vi "Calc Increment_modded.vi"(1 "desired font(Application)":T5(ring)=enum."Application Font", 2 "scale definition":T2={"coordinate 1"=5, "value 1"=5.0, "coordinate 2"=5, "value 2"=5.0, "log"=FALSE, "fmt and prec"={"format"=enum."Hex", "precision"=0}} {"value 2" format="%0.2f"; "value 1" format="%0.2f"}, 3 "scale attributes":T3={"horizontal"=TRUE, "left/top"=FALSE, "draw bar"=FALSE, "line color"=0, "text color"=0}, 5 "[user-specified font]":T4) -> (6 "start":dbl format="%0.2f", 7 "increment":dbl format="%0.2f", 9 "text size":i16)   [LabVIEW 2018]
uses:
  fmt_prec_modded.ctl
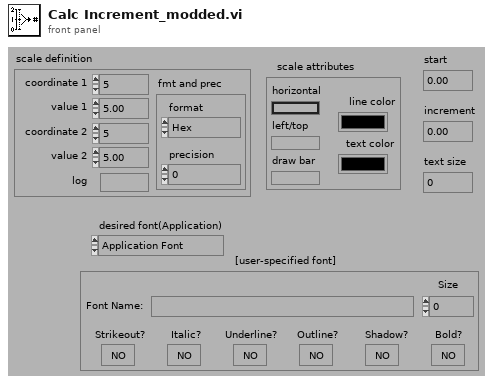
[diagram p1: front panel]
types:
  T1 = typedef "fmt_prec_modded.ctl" = cluster{"format":enum8{"Decimal", "Scientific", "Engineering", "Binary", "Octal", "Hex", "Timestamp"}, "precision":u8}
  T2 = cluster{"coordinate 1":i16, "value 1":dbl, "coordinate 2":i16, "value 2":dbl, "log":bool, "fmt and prec":T1}
  T3 = cluster{"horizontal":bool, "left/top":bool, "draw bar":bool, "line color":u32, "text color":u32}
  T4 = cluster{"Font Name:":string, "Size":i16, "Strikeout?":bool, "Italic?":bool, "Underline?":bool, "Outline?":bool, "Shadow?":bool, "Bold?":bool}
  T5 = enum16{"User-specified Font", "Application Font", "System Font", "Dialog Font"}
  T6 = cluster{"left":i16, "top":i16, "right":i16, "bottom":i16}
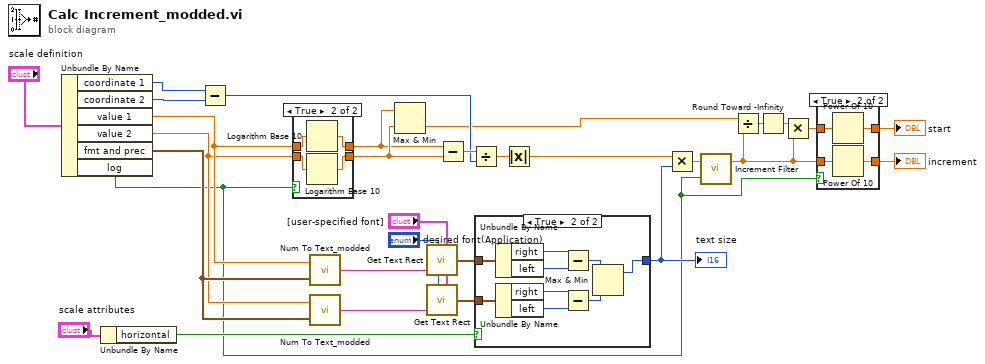
[diagram p0: block diagram]
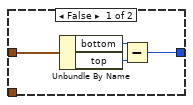
[diagram p4: hidden frame]
diagram:
  n1 = Unbundle By Name("scale definition") -> ("coordinate 1"=w14:i16, "coordinate 2"=w15:i16, "value 1"=w8:dbl, "value 2"=w7:dbl, "fmt and prec"=w28:T1, "log"=w1:bool)
  n2 = Unbundle By Name("scale attributes") -> ("horizontal"=w23:bool)
  n3 = Subtract(x=w14, y=w15) -> (x-y=w16:i16)
  n4 = case shown="True" w1 {
    tunnel: w8 -> [w32 w35]
    tunnel: [w32 w34] -> w10
    tunnel: w7 -> [w31 w36]
    tunnel: [w31 w33] -> w11
    frame False {
    }
    frame True {
      n5 = Logarithm Base 10(1:w35) -> (0:w34:dbl)
      n6 = Logarithm Base 10(1:w36) -> (0:w33:dbl)
    }
  }
  n7 = call "Num To Text_modded.vi"("fmt and prec"=w28, "number"=w8) -> ("numeric string"=w30:string)
  n8 = call "Num To Text_modded.vi"("fmt and prec"=w28, "number"=w7) -> ("numeric string"=w27:string)
  n9 = Max & Min(x=w10, y=w11) -> (min(x,y)=w9:dbl)  [unwired: 1 out]
  n10 = call <vilib>:"Get Text Rect.vi"("desired font(Application)"="desired font(Application)", "text"=w30, "[user-specified font]"="[user-specified font]") -> ("rect"=w21:T6)  [unwired: 6 in]
  n11 = call <vilib>:"Get Text Rect.vi"("desired font(Application)"="desired font(Application)", "text"=w27, "[user-specified font]"="[user-specified font]") -> ("rect"=w22:T6)  [unwired: 6 in]
  n12 = Subtract(x=w10, y=w11) -> (x-y=w18:dbl)
  n13 = Divide(x=w18, y=w16) -> (x/y=w20:dbl)
  n14 = case shown="True" w23 {
    tunnel: w22 -> [_ w48]
    tunnel: w21 -> [w38 w49]
    tunnel: [w37 w41] -> w17
    frame False {
      n15 = Unbundle By Name(w38) -> ("bottom"=w39:i16, "top"=w40:i16)
      n16 = Subtract(x=w39, y=w40) -> (x-y=w37:i16)
    }
    frame True {
      n17 = Unbundle By Name(w49) -> ("right"=w44:i16, "left"=w45:i16)
      n18 = Unbundle By Name(w48) -> ("right"=w47:i16, "left"=w46:i16)
      n19 = Subtract(x=w44, y=w45) -> (x-y=w42:i16)
      n20 = Subtract(x=w47, y=w46) -> (x-y=w43:i16)
      n21 = Max & Min(x=w42, y=w43) -> (max(x,y)=w41:i16)  [unwired: 1 out]
    }
  }
  "text size" <- w17
  n22 = Absolute Value(x=w20) -> (abs(x)=w19:dbl)
  n23 = Multiply(x=w19, y=w17) -> (x*y=w2:dbl)
  n24 = call <vilib>:"Increment Filter.vi"("log?(F)"=w1, "initial increment"=w2) -> ("nice increment"=w5:dbl)  [unwired: 1 in]
  n25 = Divide(x=w9, y=w5) -> (x/y=w13:dbl)
  n26 = Round Toward -Infinity(1:w13) -> (0:w12:dbl)
  n27 = Multiply(x=w12, y=w5) -> (x*y=w4:dbl)
  n28 = case shown="True" w1 {
    tunnel: w5 -> [w51 w55]
    tunnel: [w51 w54] -> w6
    tunnel: w4 -> [w50 w53]
    tunnel: [w50 w52] -> w3
    frame False {
    }
    frame True {
      n29 = Power Of 10(x=w53) -> (10^x=w52:dbl)
      n30 = Power Of 10(x=w55) -> (10^x=w54:dbl)
    }
  }
  "increment" <- w6
  "start" <- w3
